vi "checkTimeout.vi"(8 "error in (no error)":errorcluster, 10 "ElectrometerController in":refnum<class "ElectrometerController.lvclass">, 11 "ManualReadingState in":refnum<class "ManualReadingState.lvclass">) -> (0 "error out":errorcluster, 1 "timeout?":bool, 2 "ElectrometerController out":refnum<class "ElectrometerController.lvclass">, 3 "ManualReadingState out":refnum<class "ManualReadingState.lvclass">)   [LabVIEW 2016, in "ManualReadingState.lvclass"]
uses:
  ManualReadingState.lvclass
  ElectrometerController/ElectrometerController.lvclass
  Electrometer.lvclass
  ElectrometerConfiguration/ElectrometerInternalConfiguration.lvclass
  State.lvclass
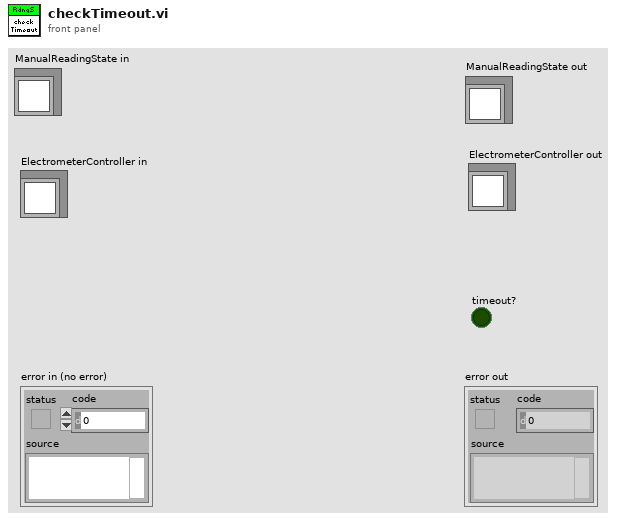
[diagram p1: front panel]
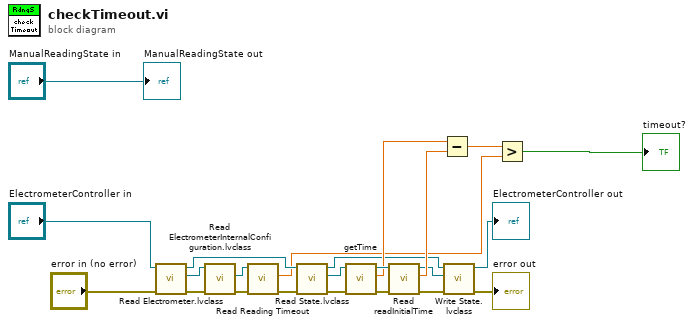
[diagram p0: block diagram]
diagram:
  n1 = call-dynamic "Read Electrometer.lvclass.vi"("error in (no error)"="error in (no error)", "ElectrometerController in"="ElectrometerController in") -> ("error out"=w19:errorcluster, "Electrometer.lvclass"=w22:refnum<class "Electrometer.lvclass">, "ElectrometerController out"=w15:refnum<class "ElectrometerController.lvclass">)  [unwired: 7 in]
  n2 = call-dynamic "Read ElectrometerInternalConfiguration.lvclass.vi"("error in (no error)"=w19, "Electrometer in"=w22) -> ("error out"=w20:errorcluster, "ElectrometerInternalConfiguration.lvclass"=w21:refnum<class "ElectrometerInternalConfiguration.lvclass">)  [unwired: 7 in, 1 out]
  n3 = call-dynamic "Read Reading Timeout.vi"("error in (no error)"=w20, "ElectrometerInternalConfiguration in"=w21) -> ("error out"=w14:errorcluster, "Reading Timeout"=w7:dbl)  [unwired: 7 in, 1 out]
  n4 = call-dynamic "Read State.lvclass.vi"("error in (no error)"=w14, "ElectrometerController in"=w15) -> ("error out"=w12:errorcluster, "State.lvclass"=w13:refnum<class "State.lvclass">, "ElectrometerController out"=w9:refnum<class "ElectrometerController.lvclass">)  [unwired: 7 in]
  n5 = call-dynamic "getTime.vi"("error in (no error)"=w12, "State in"=w13) -> ("error out"=w18:errorcluster, "relative seconds"=w17:dbl, "State out"=w23:refnum<class "State.lvclass">)  [unwired: 7 in]
  n6 = call-dynamic "Read readInitialTime.vi"("error in (no error)"=w18, "State in"=w23) -> ("error out"=w11:errorcluster, "readInitialTime"=w16:dbl, "State out"=w10:refnum<class "State.lvclass">)  [unwired: 7 in]
  n7 = Subtract(x=w17, y=w16) -> (x-y=w8:dbl)
  n8 = call-dynamic "Write State.lvclass.vi"("error in (no error)"=w11, "State.lvclass"=w10, "ElectrometerController in"=w9) -> ("error out"=→"error out":errorcluster, "ElectrometerController out"=→"ElectrometerController out":refnum<class "ElectrometerController.lvclass">)  [unwired: 7 in]
  n9 = Greater?(x=w8, y=w7) -> (0:→"timeout?":bool)
  "ManualReadingState out" <- "ManualReadingState in"
